vi "Sub05_MatlabFileBuilder.vi"(5 "Select line style":string(combo), 6 "Ball touch color":u32(colorbox), 7 "appended array":T2(array[cluster]), 8 "error in (no error)":errorcluster, 9 "Band touch color":u32(colorbox), 10 "CommandInfo":T1, 11 "Select sequence":string) -> (0 "error out":errorcluster, 3 "String":string)   [LabVIEW 2019]
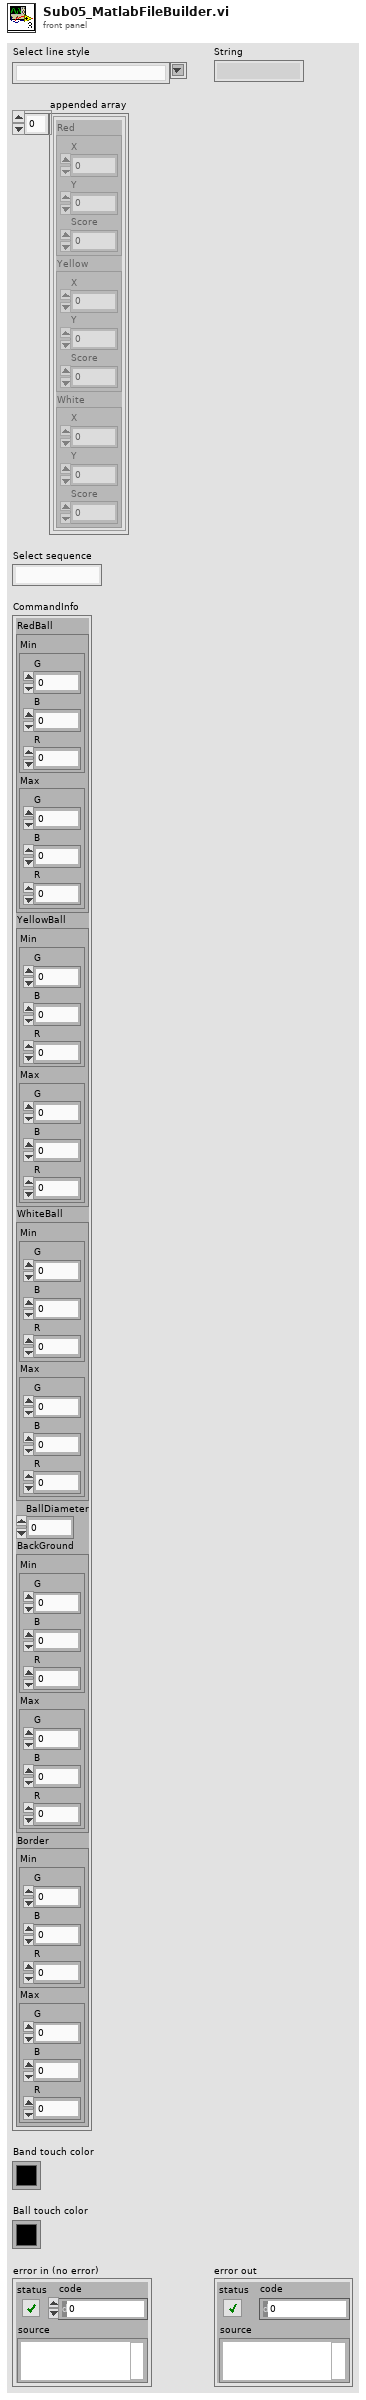
[diagram p1: front panel]
types:
  T1 = cluster{"RedBall":cluster{"Min":cluster{"G":u32, "B":u32, "R":u32}, "Max":cluster{"G":u32, "B":u32, "R":u32}}, "YellowBall":cluster{"Min":cluster{"G":u32, "B":u32, "R":u32}, "Max":cluster{"G":u32, "B":u32, "R":u32}}, "WhiteBall":cluster{"Min":cluster{"G":u32, "B":u32, "R":u32}, "Max":cluster{"G":u32, "B":u32, "R":u32}}, "BallDiameter":u32, "BackGround":cluster{"Min":cluster{"G":u32, "B":u32, "R":u32}, "Max":cluster{"G":u32, "B":u32, "R":u32}}, "Border":cluster{"Min":cluster{"G":u32, "B":u32, "R":u32}, "Max":cluster{"G":u32, "B":u32, "R":u32}}}
  T2 = cluster{"Red":cluster{"X":u32, "Y":u32, "Score":u32}, "Yellow":cluster{"X":u32, "Y":u32, "Score":u32}, "White":cluster{"X":u32, "Y":u32, "Score":u32}}[]
  T3 = cluster{"Min":cluster{"G":u32, "B":u32, "R":u32}, "Max":cluster{"G":u32, "B":u32, "R":u32}}
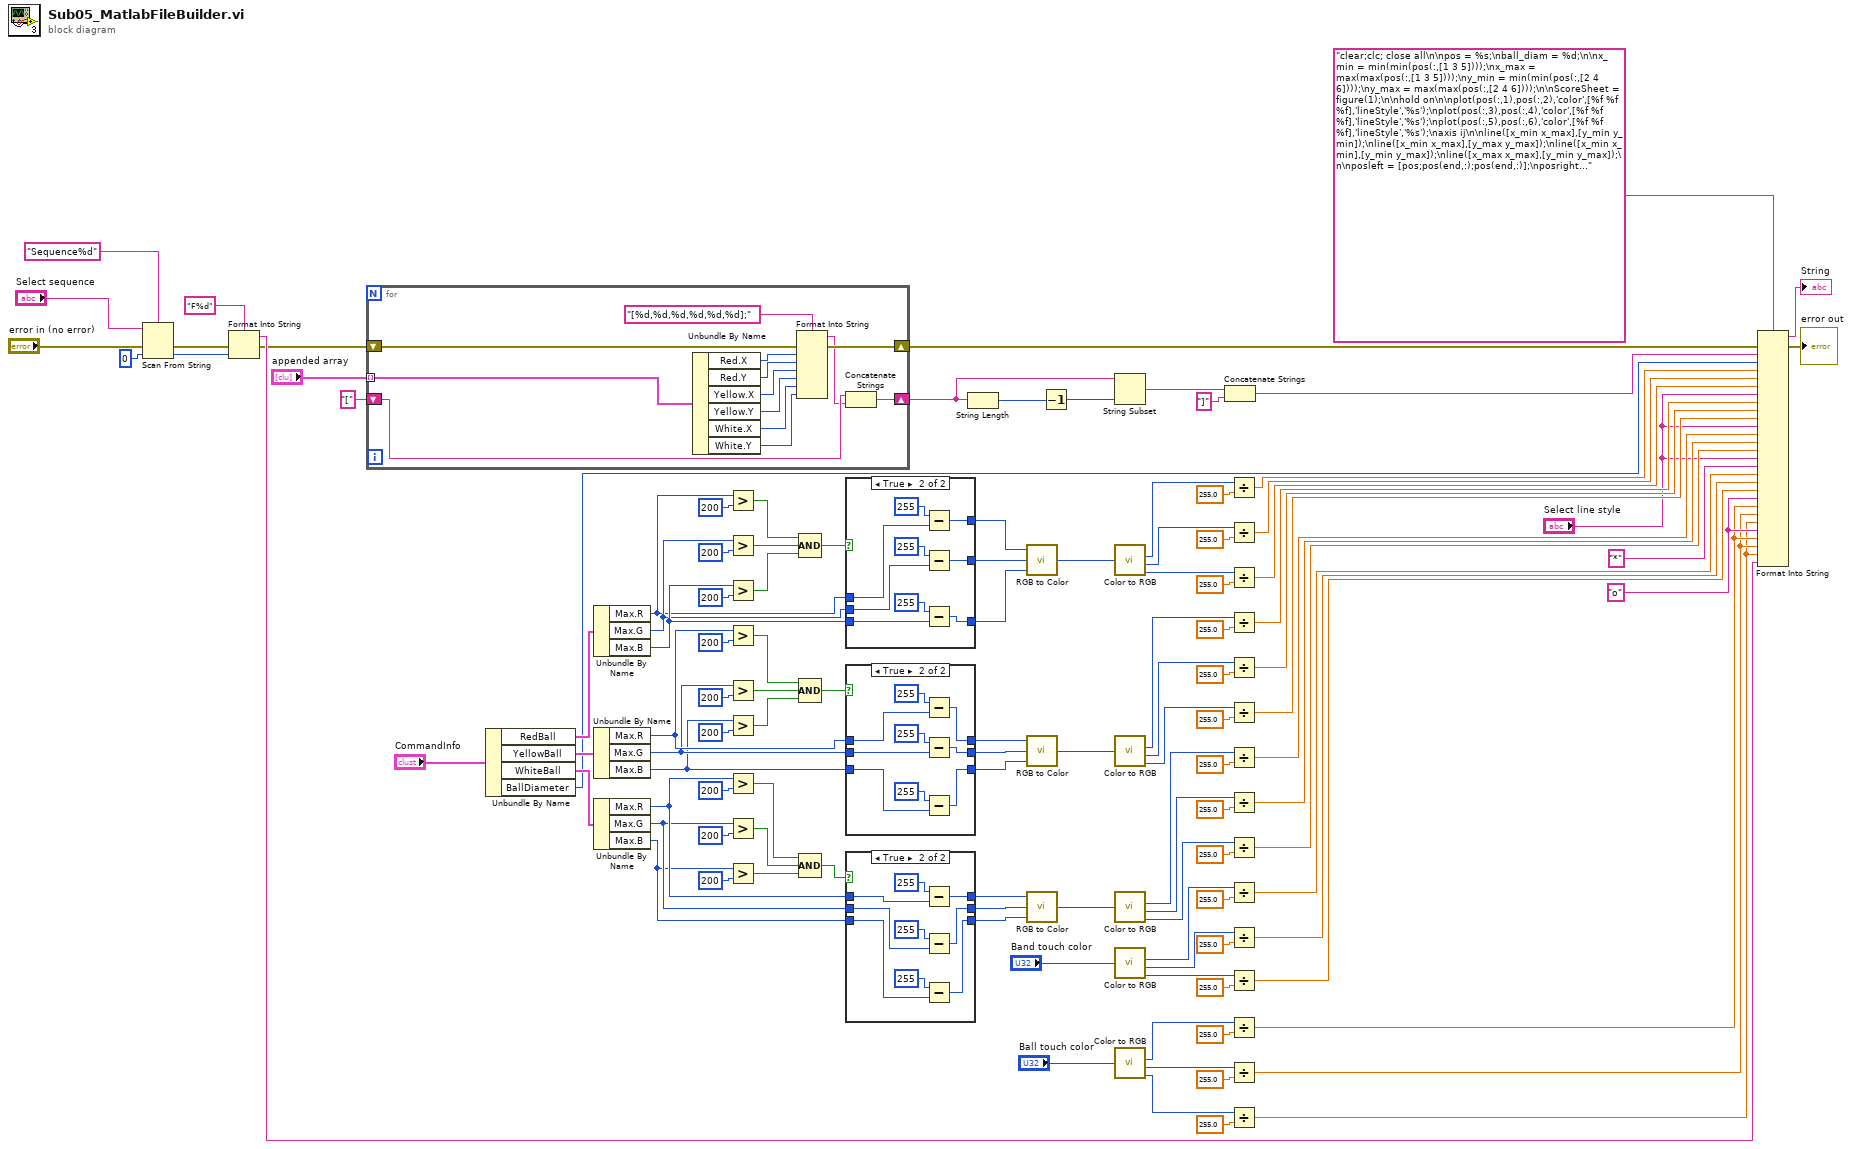
[diagram p0: block diagram]
diagram:
  w42 = "o" ("input 34")
  n1 = Scan From String(format string="Sequence%d", input string="Select sequence", error in="error in (no error)", default 1=0 ("default value 1")) -> (error out=w36:errorcluster, output 1=w35:i32)  [unwired: 1 in, 2 out]
  n2 = Format Into String(format string="F%d", error in=w36, w35) -> (resulting string=w118:string, error out=w37:errorcluster)  [unwired: 1 in]
  n3 = for {
    tunnel: "appended array" -> [w131] mode=indexing
    shift-right: [w123] -> w93
    shift-left: "[" -> [w124]
    shift-right: [w121] -> w49
    shift-left: w37 -> [w122]
    n4 = Unbundle By Name(w131) -> ("Red.X"=w130:u32, "Red.Y"=w129:u32, "Yellow.X"=w128:u32, "Yellow.Y"=w127:u32, "White.X"=w126:u32, "White.Y"=w125:u32)
    n5 = Format Into String(format string="[%d,%d,%d,%d,%d,%d];" ("initial string"), error in=w122, w130, w129, w128, w127, w126, w125) -> (resulting string=w120:string, error out=w121:errorcluster)  [unwired: 1 in]
    n6 = Concatenate Strings(w124, w120) -> (w123:string)
  }
  n7 = Unbundle By Name("CommandInfo") -> ("RedBall"=w38:T3, "YellowBall"=w110:T3, "WhiteBall"=w114:T3, "BallDiameter"=w24:u32)
  n8 = Unbundle By Name(w38) -> ("Max.R"=w101:u32, "Max.G"=w102:u32, "Max.B"=w103:u32)
  n9 = Unbundle By Name(w110) -> ("Max.R"=w22:u32, "Max.G"=w21:u32, "Max.B"=w20:u32)
  n10 = Unbundle By Name(w114) -> ("Max.R"=w15:u32, "Max.G"=w14:u32, "Max.B"=w13:u32)
  n11 = Greater?(x=w101, y=u32 200) -> (0:w97:bool)
  n12 = Greater?(x=w102, y=u32 200) -> (0:w98:bool)
  n13 = Greater?(x=w103, y=u32 200) -> (0:w99:bool)
  n14 = Greater?(x=w22, y=u32 200) -> (0:w107:bool)
  n15 = Greater?(x=w21, y=u32 200) -> (0:w108:bool)
  n16 = Greater?(x=w20, y=u32 200) -> (0:w109:bool)
  n17 = Greater?(x=w15, y=u32 200) -> (0:w111:bool)
  n18 = Greater?(x=w14, y=u32 200) -> (0:w112:bool)
  n19 = Greater?(x=w13, y=u32 200) -> (0:w113:bool)
  n20 = Compound Arithmetic op=AND(w97, w98, w99) -> (w100:bool)
  n21 = Compound Arithmetic op=AND(w107, w108, w109) -> (w23:bool)
  n22 = Compound Arithmetic op=AND(w111, w112, w113) -> (w16:bool)
  n23 = case shown="True" w100 {
    tunnel: w101 -> [w134 w143]
    tunnel: w102 -> [w133 w142]
    tunnel: w103 -> [w132 w141]
    tunnel: [w134 w139] -> w104
    tunnel: [w133 w138] -> w105
    tunnel: [w132 w137] -> w106
    frame False {
    }
    frame True {
      n24 = Subtract(x=u32 255, y=w143) -> (x-y=w139:u32)
      n25 = Subtract(x=u32 255, y=w142) -> (x-y=w138:u32)
      n26 = Subtract(x=u32 255, y=w141) -> (x-y=w137:u32)
    }
  }
  n27 = case shown="True" w23 {
    tunnel: w22 -> [w146 w155]
    tunnel: w21 -> [w145 w154]
    tunnel: w20 -> [w144 w153]
    tunnel: [w146 w151] -> w19
    tunnel: [w145 w150] -> w18
    tunnel: [w144 w149] -> w17
    frame False {
    }
    frame True {
      n28 = Subtract(x=u32 255, y=w155) -> (x-y=w151:u32)
      n29 = Subtract(x=u32 255, y=w154) -> (x-y=w150:u32)
      n30 = Subtract(x=u32 255, y=w153) -> (x-y=w149:u32)
    }
  }
  n31 = case shown="True" w16 {
    tunnel: w15 -> [w158 w167]
    tunnel: w14 -> [w157 w166]
    tunnel: w13 -> [w156 w165]
    tunnel: [w158 w163] -> w12
    tunnel: [w157 w162] -> w11
    tunnel: [w156 w161] -> w10
    frame False {
    }
    frame True {
      n32 = Subtract(x=u32 255, y=w167) -> (x-y=w163:u32)
      n33 = Subtract(x=u32 255, y=w166) -> (x-y=w162:u32)
      n34 = Subtract(x=u32 255, y=w165) -> (x-y=w161:u32)
    }
  }
  n35 = String Length(string=w93) -> (length=w95:i32)
  n36 = call <vilib>:"RGB to Color.vi"("B"=w106, "G"=w105, "R"=w104) -> ("Color"=w115:u32)
  n37 = call <vilib>:"RGB to Color.vi"("B"=w17, "G"=w18, "R"=w19) -> ("Color"=w116:u32)
  n38 = call <vilib>:"RGB to Color.vi"("B"=w10, "G"=w11, "R"=w12) -> ("Color"=w117:u32)
  n39 = Decrement(x=w95) -> (x-1=w94:i32)
  n40 = String Subset(string=w93, length (rest)=w94) -> (substring=w92:string)  [unwired: 1 in]
  n41 = call <vilib>:"Color to RGB.vi"("Color"=w115) -> ("R"=w79:u8, "G"=w78:u8, "B"=w77:u8)  [unwired: 1 out]
  n42 = call <vilib>:"Color to RGB.vi"("Color"=w116) -> ("R"=w76:u8, "G"=w75:u8, "B"=w74:u8)  [unwired: 1 out]
  n43 = call <vilib>:"Color to RGB.vi"("Color"=w117) -> ("R"=w73:u8, "G"=w72:u8, "B"=w71:u8)  [unwired: 1 out]
  n44 = call <vilib>:"Color to RGB.vi"("Color"="Band touch color") -> ("R"=w58:u8, "G"=w57:u8, "B"=w56:u8)  [unwired: 1 out]
  n45 = call <vilib>:"Color to RGB.vi"("Color"="Ball touch color") -> ("R"=w52:u8, "G"=w51:u8, "B"=w50:u8)  [unwired: 1 out]
  n46 = Concatenate Strings(w92, "]" ("string")) -> (w89:string)
  n47 = Divide(x=w79, y=255.0) -> (x/y=w70:dbl)
  n48 = Divide(x=w78, y=255.0) -> (x/y=w69:dbl)
  n49 = Divide(x=w77, y=255.0) -> (x/y=w68:dbl)
  n50 = Divide(x=w76, y=255.0) -> (x/y=w67:dbl)
  n51 = Divide(x=w75, y=255.0) -> (x/y=w66:dbl)
  n52 = Divide(x=w74, y=255.0) -> (x/y=w65:dbl)
  n53 = Divide(x=w73, y=255.0) -> (x/y=w64:dbl)
  n54 = Divide(x=w72, y=255.0) -> (x/y=w63:dbl)
  n55 = Divide(x=w71, y=255.0) -> (x/y=w62:dbl)
  n56 = Divide(x=w58, y=255.0) -> (x/y=w45:dbl)
  n57 = Divide(x=w57, y=255.0) -> (x/y=w44:dbl)
  n58 = Divide(x=w56, y=255.0) -> (x/y=w43:dbl)
  n59 = Divide(x=w52, y=255.0) -> (x/y=w41:dbl)
  n60 = Divide(x=w51, y=255.0) -> (x/y=w40:dbl)
  n61 = Divide(x=w50, y=255.0) -> (x/y=w39:dbl)
  n62 = Format Into String(format string="clear;clc; close all\n\npos = %s;\nball_diam = %d;\n\nx_min = min(min(pos(:,[1 3 5])));\nx_max = max(max(pos(:,[1 3 5])));\ny_min = min(min(pos(:,[2 4 6])));\ny_max = max(max(pos(:,[2 4 6])));\n\nScoreSheet = figure(1);\n\nhold on\n\nplot(pos(:,1),pos(:,2),'color',[%f %f %f],'lineStyle','%s');\nplot(pos(:,3),pos(:,4),'color',[%f %f %f],'lineStyle','%s');\nplot(pos(:,5),pos(:,6),'color',[%f %f %f],'lineStyle','%s');\naxis ij\n\nline([x_min x_max],[y_min y_min]);\nline([x_min x_max],[y_max y_max]);\nline([x_min x_min],[y_min y_max]);\nline([x_max x_max],[y_min y_max]);\n\nposleft = [pos;pos(end,:);pos(end,:)];\nposright = [pos(1,:);pos(1,:);pos];\npos = [pos(1,:);pos;pos(end,:)];\n\nvel = (posright-posleft)/2;\nacc = (posright-2*pos+posleft)/4;\n\ndist(1) = floor(sum(sqrt(vel(2:end-1,1).^2+vel(2:end-1,2).^2)));\ndist(2) = floor(sum(sqrt(vel(2:end-1,3).^2+vel(2:end-1,4).^2)));\ndist(3) = floor(sum(sqrt(vel(2:end-1,5).^2+vel(2:end-1,6).^2)));\n\nvelleft=[vel(2:end,:);vel(end,:)];\nvelright=[vel(1,:);vel(1:end-1,:)];\n\nmoving(:,1) = (pos(:,1)-pos(1,1)).^2 + (pos(:,2)-pos(1,2)).^2 >= 100;\nmoving(:,2) = (pos(:,3)-pos(1,3)).^2 + (pos(:,4)-pos(1,4)).^2 >= 100;\nmoving(:,3) = (pos(:,5)-pos(1,5)).^2 + (pos(:,6)-pos(1,6)).^2 >= 100;\n\n[player_ball,~] = find(moving',1);\n\nif player_ball == 1\n    player='red';\n    ball_a = 2;\n    ball_b = 3;\nelseif player_ball == 2\n    player='yellow';\n    ball_a = 1;\n    ball_b = 3;\nelse\n    player='white';\n    player_ball = 3;\n    ball_a = 1;\n    ball_b = 2;\nend\n\nvel_comp = sqrt(max(vel(:,2*player_ball-1).^2+vel(:,2*player_ball).^2,max(velleft(:,2*player_ball-1).^2+velleft(:,2*player_ball).^2,velright(:,2*player_ball-1).^2+velright(:,2*player_ball).^2)));\n\nvel_comp_a = ball_diam + sqrt(max((vel(:,2*player_ball-1)-vel(:,2*ball_a-1)).^2+(vel(:,2*player_ball)-vel(:,2*ball_a)).^2,max((velleft(:,2*player_ball-1)-velleft(:,2*ball_a-1)).^2+(velleft(:,2*player_ball)-velleft(:,2*ball_a)).^2,(velright(:,2*player_ball-1)-velright(:,2*ball_a-1)).^2+(velright(:,2*player_ball)-velright(:,2*ball_a)).^2)));\nvel_comp_b = ball_diam + sqrt(max((vel(:,2*player_ball-1)-vel(:,2*ball_b-1)).^2+(vel(:,2*player_ball)-vel(:,2*ball_b)).^2,max((velleft(:,2*player_ball-1)-velleft(:,2*ball_b-1)).^2+(velleft(:,2*player_ball)-velleft(:,2*ball_b)).^2,(velright(:,2*player_ball-1)-velright(:,2*ball_b-1)).^2+(velright(:,2*player_ball)-velright(:,2*ball_b)).^2)));\n\nband_touch_left = velleft(:,2*player_ball-1) < 0 & velright(:,2*player_ball-1) > 0 & (pos(:,2*player_ball-1)-x_min) <= vel_comp;\nband_touch_right = velleft(:,2*player_ball-1) > 0 & velright(:,2*player_ball-1) < 0 & (-pos(:,2*player_ball-1)+x_max) <= vel_comp;\nband_touch_up = velleft(:,2*player_ball) < 0 & velright(:,2*player_ball) > 0 & (pos(:,2*player_ball)-y_min) <= vel_comp;\nband_touch_down = velleft(:,2*player_ball) > 0 & velright(:,2*player_ball) < 0 & (-pos(:,2*player_ball)+y_max) <= vel_comp;\nball_touch_a = (abs(acc(:,2*player_ball-1)) > 0 | abs(acc(:,2*player_ball)) > 0) & (abs(acc(:,2*ball_a-1)) > 0 | abs(acc(:,2*ball_a)) > 0) & ((pos(:,2*player_ball-1)-pos(:,2*ball_a-1)).^2 + (pos(:,2*player_ball)-pos(:,2*ball_a)).^2) < vel_comp_a.^2;\nball_touch_b = (abs(acc(:,2*player_ball-1)) > 0 | abs(acc(:,2*player_ball)) > 0) & (abs(acc(:,2*ball_b-1)) > 0 | abs(acc(:,2*ball_b)) > 0) & ((pos(:,2*player_ball-1)-pos(:,2*ball_b-1)).^2 + (pos(:,2*player_ball)-pos(:,2*ball_b)).^2) < vel_comp_b.^2;\n\nband_touch_left_right = [band_touch_left(1);band_touch_left(1:end-1)];\nband_touch_right_right = [band_touch_right(1);band_touch_right(1:end-1)];\nband_touch_up_right = [band_touch_up(1);band_touch_up(1:end-1)];\nband_touch_down_right = [band_touch_down(1);band_touch_down(1:end-1)];\nball_touch_a_right = [ball_touch_a(1);ball_touch_a(1:end-1)];\nball_touch_b_right = [ball_touch_b(1);ball_touch_b(1:end-1)];\n\nband_touch_left(band_touch_left & band_touch_left_right) = 0;\nband_touch_right(band_touch_right & band_touch_right_right) = 0;\nband_touch_up(band_touch_up & band_touch_up_right) = 0;\nband_touch_down(band_touch_down & band_touch_down_right) = 0;\nball_touch_a(ball_touch_a & ball_touch_a_right) = 0;\nball_touch_b(ball_touch_b & ball_touch_b_right) = 0;\n\nband_touch=find(band_touch_left | band_touch_right | band_touch_up | band_touch_down);\nball_touch_a = find(ball_touch_a);\nball_touch_b = find(ball_touch_b);\n\nplot(pos(band_touch,2*player_ball-1),pos(band_touch,2*player_ball),'Marker','%s','lineStyle','none','color',[%f %f %f]);\nplot(pos(ball_touch_a,2*player_ball-1),pos(ball_touch_a,2*player_ball),'Marker','%s','lineStyle','none','color',[%f %f %f]);\nplot(pos(ball_touch_b,2*player_ball-1),pos(ball_touch_b,2*player_ball),'Marker','%s','lineStyle','none','color',[%f %f %f]);\n\nwin = 0;\n\nif numel(ball_touch_a) && numel(ball_touch_b) && numel(band_touch)>=3\n    if max(ball_touch_a) < min(ball_touch_b)\n        band_touch = band_touch(band_touch>max(ball_touch_a) & band_touch<min(ball_touch_b));\n        if numel(band_touch)>=3\n            win = 1;\n        end\n    else\n        band_touch = band_touch(band_touch>max(ball_touch_b) & band_touch<min(ball_touch_a));\n        if numel(band_touch)>=3\n            win = 1;\n        end\n    end\nend\n\nif numel(ball_touch_a) && numel(ball_touch_b)\n    balls_touched_t = \"2 balls touched\";\nelseif numel(ball_touch_a) || numel(ball_touch_b)\n    balls_touched_t = \"1 ball touched\";\nelse\n    balls_touched_t = \"No ball touched\";\nend\n\nif numel(band_touch) >= 2\n    band_touched_t = sprintf(\"\\%d bands touched\",numel(band_touch));\nelseif numel(band_touch) == 1\n    band_touched_t = \"1 band touched\";\nelse\n    band_touched_t = \"No band touched\";\nend\n\nif win\n    win_mess = \"You won. You're wonderful <3\";\nelse\n    win_mess = \"You lost. You litte shit.\";\nend\n\ntext_to_display = {sprintf(\"Scores for player \\%s\",player),balls_touched_t,band_touched_t,sprintf(\"dist(r) = \\%dpx\",dist(1)),sprintf(\"dist(y) = \\%dpx\",dist(2)),sprintf(\"dist(w) = \\%dpx\",dist(3)),win_mess};\nx_text = x_min + [1 13 13 1 7 13 1]*(x_max-x_min)/18;\ny_text = y_max + [14 14 43 72 72 72 43];\ntext(x_text,y_text,text_to_display);\n\ntime_t = floor(clock);\nscoresheet_title = sprintf('Scores Sheet - %s - \\%s \\%dh\\%dmin\\%ds',date,time_t(4:6));\nsgtitle(scoresheet_title)\n\naxis([x_min-5 x_max+5 y_min-5 y_max+100]);\nset(gca,'visible','off');\nset(gca,'xtick',[]);\n\nset(gcf, 'PaperUnits', 'centimeters', 'Units', 'centimeters');\nset(gcf, 'PaperSize', [29.7 21]);\nset(gcf, 'Position', [0.5 0.5 28.7 20]);\n\nsaveas(ScoreSheet,'ScoreSheet','pdf');\nopen('ScoreSheet.pdf');\n\nclc;clear;\n\nreturn", error in=w49, w89, w24, w70, w69, w68, "Select line style", w67, w66, w65, "Select line style", w64, w63, w62, "Select line style", "*" ("input 18"), w45, w44, w43, w42, w41, w40, w39, w42, w41, w40, w39, w118) -> (resulting string=→"String":string, error out=→"error out":errorcluster)  [unwired: 1 in]
